vi "Get Input.vi"() -> (3 "Input":string)   [LabVIEW 2025, in "AOC.lvlib"]
uses:
  AOC.lvlib
  <vilib>/Utility/error.llb/whitespace.ctl
  <vilib>/Utility/error.llb/Trim Whitespace One-Sided.vi
  <vilib>/httpClient/LabVIEWHTTPClient.lvlib
  <userlib>/_OpenG.lib/appcontrol/appcontrol.llb/openg_application_control.lvlib
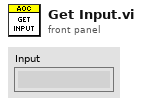
[diagram p1: front panel]
types:
  T1 = enum16{"open", "replace", "create", "open or create", "replace or create", "replace or create with confirmation"}
  T2 = typedef "whitespace.ctl" = u16
  T3 = typedef "LabVIEWHTTPClient.lvlib/ClientHandle.ctl" = refnum<k1>
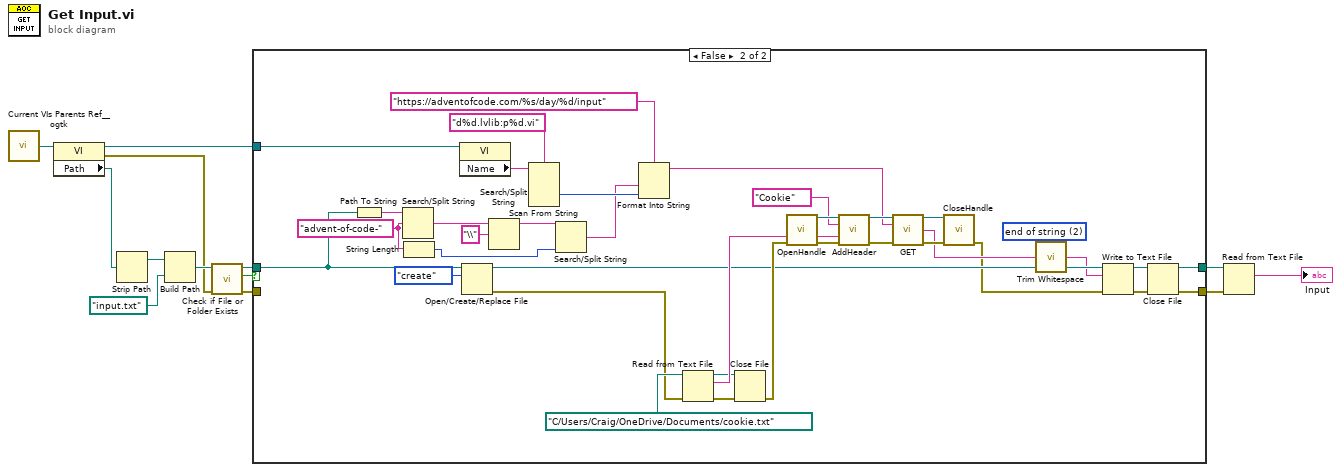
[diagram p0: block diagram]
diagram:
  n1 = call <userlib>:"Current VIs Parents Ref__ogtk.vi"() -> ("Calling VI's Reference"=w13:refnum<vi>)  [unwired: 2 in]
  n2 = property class="VI"(reference=w13) -> (reference out=w7:refnum<vi>, error out=w1:errorcluster, "Path"=w12:path)  [unwired: 1 in]
  n3 = Strip Path(path=w12) -> (stripped path=w10:path)  [unwired: 1 out]
  n4 = Build Path(base path=w10, name or relative path=path "input.txt") -> (appended path=w11:path)
  n5 = call <vilib>:"Check if File or Folder Exists.vi"("error in (no error)"=w1, "path"=w11) -> ("error out"=w2:errorcluster, "file or folder exists?"=w8:bool, "dup path"=w6:path)  [unwired: 7 in]
  n6 = case shown="False" w8 {
    tunnel: w7 -> [_ w35]
    tunnel: w6 -> [w15 w23]
    tunnel: [w15 w29] -> w5
    tunnel: [w14 w24] -> w3
    tunnel: w2 -> [w14 _]
    frame True {
    }
    frame False {
      w18 = "advent-of-code-" ("search string/char (-)")
      w37 = T2 2 items=["both", "start of string", "end of string"] ("location (both)")
      n7 = Path To String(path=w23) -> (string=w22:string)
      n8 = Search/Split String(string=w22, search string/char (-)=w18) -> (match + rest of string=w21:string)  [unwired: 1 in, 2 out]
      n9 = String Length(string=w18) -> (length=w17:i32)
      n10 = property class="VI"(reference=w35) -> ("Name"=w39:string)  [unwired: 1 in, 2 out]
      n11 = Open/Create/Replace File(file path (use dialog)=w23, operation (0:open)=T1."create") -> (refnum out=w31:refnum<file>, error out=w26:errorcluster)  [unwired: 4 in, 1 out]
      n12 = Search/Split String(string=w21, search string/char (-)="\\") -> (substring before match=w19:string)  [unwired: 1 in, 2 out]
      n13 = Scan From String(format string="d%d.lvlib:p%d.vi", input string=w39) -> (output 1=w38:i32)  [unwired: 5 in, 3 out]
      n14 = Search/Split String(string=w19, offset (0)=w17) -> (match + rest of string=w16:string)  [unwired: 1 in, 2 out]
      n15 = Format Into String(format string="https://adventofcode.com/%s/day/%d/input", w16, w38) -> (resulting string=w42:string)  [unwired: 2 in, 1 out]
      n16 = Read from Text File(file (use dialog)=path "C:/Users/Craig/OneDrive/Documents/cookie.txt", error in=w26) -> (refnum out=w45:refnum<file>, text=w46:string, error out=w33:errorcluster)  [unwired: 2 in, 1 out]
      n17 = Close File(refnum=w45, error in=w33) -> (error out=w32:errorcluster)  [unwired: 1 out]
      n18 = call <vilib>:"OpenHandle.vi"("error in (no error)"=w32) -> ("client handle out"=w51:T3, "error out"=w50:errorcluster)  [unwired: 13 in]
      n19 = call <vilib>:"AddHeader.vi"("client handle"=w51, "header"="Cookie", "value"=w46, "error in (no error)"=w50) -> ("client handle out"=w44:T3, "error out"=w43:errorcluster)  [unwired: 10 in]
      n20 = call <vilib>:"GET.vi"("client handle"=w44, "url"=w42, "error in (no error)"=w43) -> ("client handle out"=w41:T3, "body"=w36:string, "error out"=w40:errorcluster)  [unwired: 9 in, 1 out]
      n21 = call <vilib>:"CloseHandle.vi"("client handle"=w41, "error in (no error)"=w40) -> ("error out"=w25:errorcluster)  [unwired: 13 in]
      n22 = call <vilib>:"Trim Whitespace.vi"("string"=w36, "location (both)"=w37) -> ("trimmed string"=w27:string)
      n23 = Write to Text File(file (use dialog)=w31, text=w27, error in=w25) -> (refnum out=w30:refnum<file>, error out=w28:errorcluster)  [unwired: 1 in, 1 out]
      n24 = Close File(refnum=w30, error in=w28) -> (path=w29:path, error out=w24:errorcluster)
    }
  }
  n25 = Read from Text File(file (use dialog)=w5, error in=w3) -> (text=→"Input":string)  [unwired: 2 in, 3 out]
